vi "4.3.vi"() -> ()   [LabVIEW 2017]
panel:
  out "数值 3":dbl
  in  "x":dbl
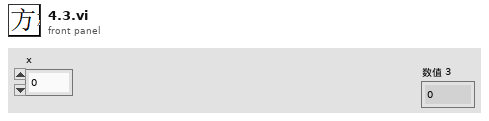
[diagram p1: front panel]
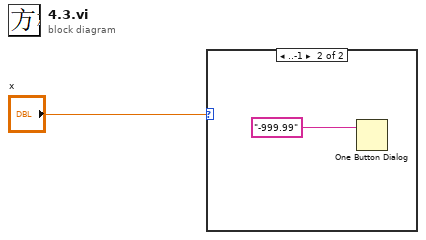
[diagram p0: block diagram]
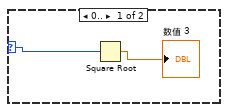
[diagram p2: hidden frame]
diagram:
  n1 = case shown="..-1" "x" {
    selector: "x" -> [w2 _]
    frame 0.. {
      n2 = Square Root(x=w2) -> (sqrt(x)=→"数值 3":dbl)
    }
    frame ..-1 {
      n3 = One Button Dialog(message="-999.99") -> ()  [unwired: 1 in, 1 out]
    }
  }
